vi "Ping ICPDAS ET7000 modules an UDP.vi"(8 "error in (no error)":errorcluster, 9 "timeout ms (100)":i32=100, 10 "Request":string="ICPDAS7188E,00\r", 11 "IP addr":string="192.168.0.1") -> (0 "error out":errorcluster, 3 "OK":bool)   [LabVIEW 2021, in "TCP.lvclass"]
uses:
  TCP.lvclass
panel:
  in  "Ring":u16(ring)
  out "Array":string[](array[string])
  # "Protocol"
  # "Version"
  # "NAME"
  # "ALIAS"
  # "LOCK"
  # "DHCP"
  # "IP"
  # "MASK"
  # "GATEWAY"
  # "MAC"
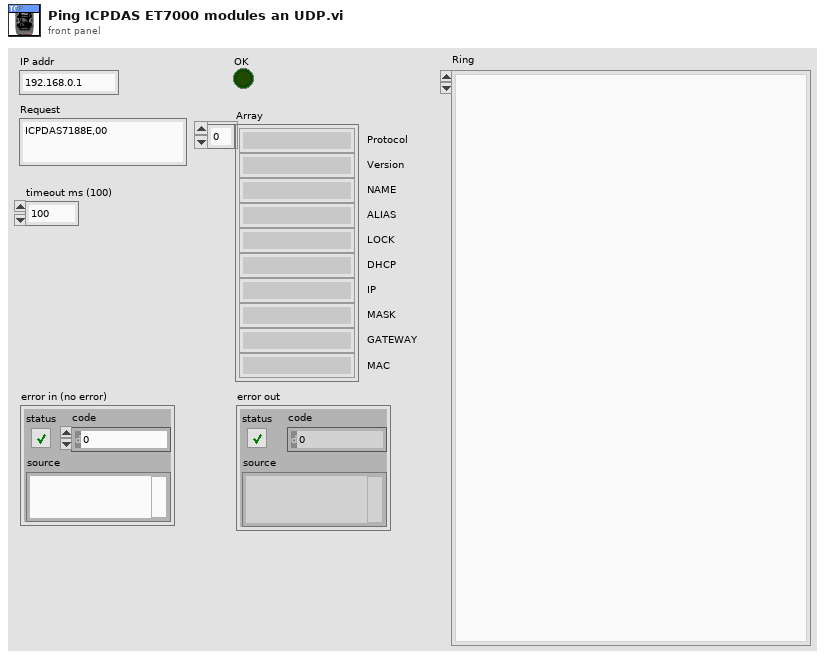
[diagram p1: front panel]
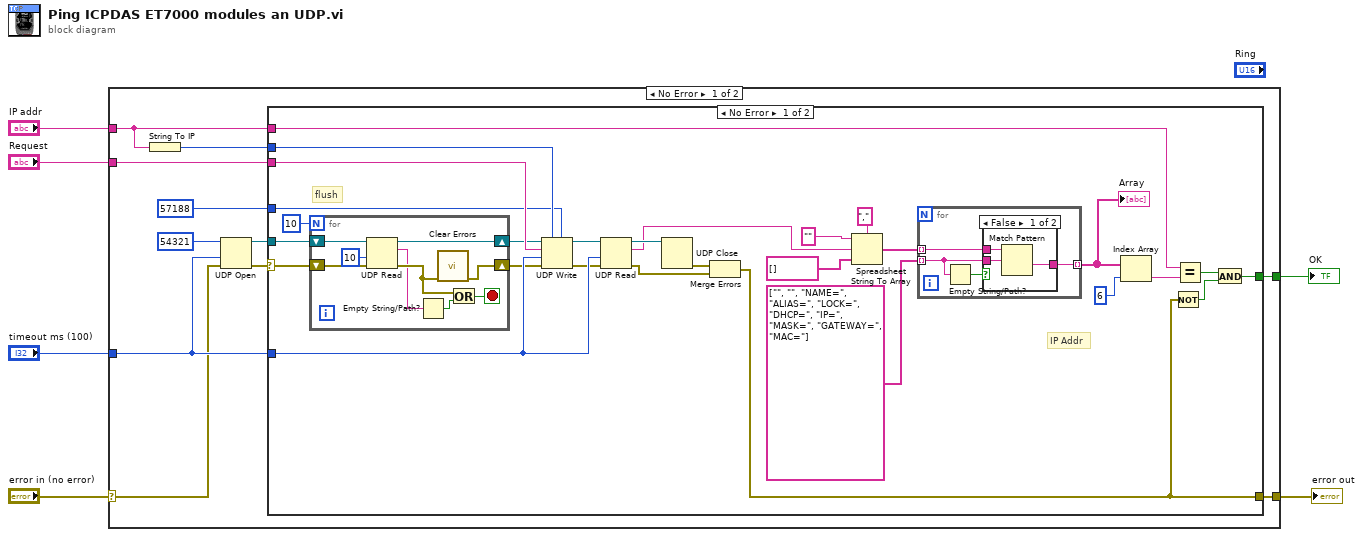
[diagram p0: block diagram]
diagram:
  n1 = case shown="No Error" "error in (no error)" {
    selector: "error in (no error)" -> [w10 w64]
    tunnel: "Request" -> [w17 _]
    tunnel: "timeout ms (100)" -> [w14 _]
    tunnel: "IP addr" -> [w12 _]
    tunnel: [w11 w64] -> w3
    tunnel: [w9 _] -> w1
    frame No Error {
      n2 = String To IP(1:w12) -> (0:w16:u32)
      n3 = UDP Open(8:w10, 9:w14, 11:u16 54321 ("port")) -> (port=w8:refnum<k16>, 0:w7:errorcluster)  [unwired: 2 in, 1 out]
      n4 = case shown="No Error" w7 {
        selector: w7 -> [w20 w63]
        tunnel: w17 -> [w42 _]
        tunnel: w16 -> [w41 _]
        tunnel: u16 57188 ("port") -> [w40 _]
        tunnel: w14 -> [w39 _]
        tunnel: w12 -> [w27 _]
        tunnel: [w25 w63] -> w11
        tunnel: [w23 _] -> w9
        tunnel: w8 -> [w22 _]
        frame No Error {
          # "flush"
          # "IP Addr"
          n5 = for {
            N: 10 -> [_]
            shift-right: [w53] -> w21
            shift-left: w22 -> [w54]
            shift-right: [w50] -> w18
            shift-left: w20 -> [w51]
            stop <- w46 stop-if-true
            n6 = UDP Read(connection ID=w54, timeout ms (25000)=10, 8:w51) -> (data out=w48:string, error out=w49:errorcluster, 3:w53:refnum<k16>)  [unwired: 1 in, 2 out]
            n7 = Empty String/Path?(string/path=w48) -> (empty?=w47:bool)
            n8 = call <vilib>:"Clear Errors.vi"("error in (no error)"=w49) -> ("error out"=w50:errorcluster)  [unwired: 5 in, 1 out]
            n9 = Or(x=w49, y=w47) -> (x .or. y?=w46:bool)
          }
          n10 = UDP Write(address=w41, port or service name=w40, connection ID=w21, data in=w42, 8:w18, 9:w39) -> (error out=w38:errorcluster, 3:w37:refnum<k16>)
          n11 = UDP Read(connection ID=w37, timeout ms (25000)=w39, 8:w38) -> (data out=w31:string, error out=w43:errorcluster, 3:w45:refnum<k16>)  [unwired: 1 in, 2 out]
          n12 = UDP Close(connection ID=w45) -> (error out=w44:errorcluster)  [unwired: 1 in, 1 out]
          n13 = Merge Errors(w44, w43) -> (w25:errorcluster)
          n14 = Spreadsheet String To Array(delimiter (Tab)=",", format string="", spreadsheet string=w31, array type (2D Dbl)=string[] []) -> (array=w32:string[])
          n15 = for {
            tunnel: string[] ["", "", "NAME=", "ALIAS=", "LOCK=", "DHCP=", "IP=", "MASK=", "GATEWAY=", "MAC="] -> [w55] mode=indexing
            tunnel: w32 -> [w58] mode=indexing
            tunnel: [w57] -> w30 mode=indexing
            n16 = Empty String/Path?(string/path=w55) -> (empty?=w56:bool)
            n17 = case shown="False" w56 {
              tunnel: w55 -> [w61 _]
              tunnel: w58 -> [w60 w62]
              tunnel: [w59 w62] -> w57
              frame False {
                n18 = Match Pattern(string=w60, regular expression=w61) -> (after substring=w59:string)  [unwired: 1 in, 3 out]
              }
              frame True {
              }
            }
          }
          "Array" <- w30
          n19 = Index Array(array=w30, index=6) -> (element=w28:string)
          n20 = Not(x=w25) -> (.not. x?=w24:bool)
          n21 = Equal?(x=w27, y=w28) -> (x = y?=w26:bool)
          n22 = And(x=w26, y=w24) -> (x .and. y?=w23:bool)
        }
        frame Error {
        }
      }
    }
    frame Error {
    }
  }
  "error out" <- w3
  "OK" <- w1
